vi "Keith 7001 Digital Out Setup.vi"(1 "channel 4 polarity":bool=TRUE, 2 "channel 4 status":bool, 3 "channel 3 polarity":bool=TRUE, 4 "channel 3 status":bool, 5 "channel 2 polarity":bool=TRUE, 6 "channel 2 status":bool, 7 "error in":T1, 8 "channel 1 polarity":bool=TRUE, 9 "channel 1 status":bool, 10 "GPIB address":string="7") -> (0 "error out":T1)   [LabVIEW 2019]
doc: "This VI for the Keithley 7001 Switch System sets the state and polarity (active high/low) of the four digital output ports."
panel:
  # "on\noff"
  # "active high\nactive low"
  # "on\noff"
  # "active high\nactive low"
  # "on\noff"
  # "active high\nactive low"
  # "on\noff"
  # "active high\nactive low"
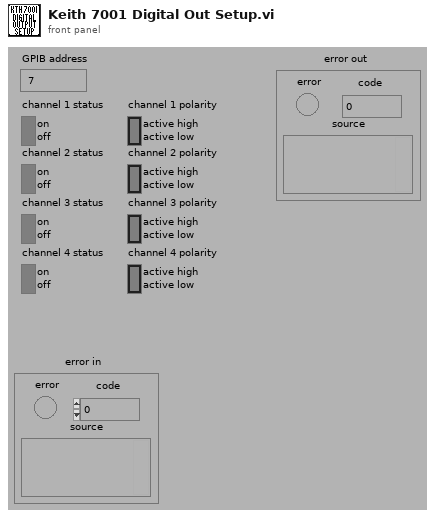
[diagram p1: front panel]
types:
  T1 = cluster{"error":bool, "code":i32, "source":string}
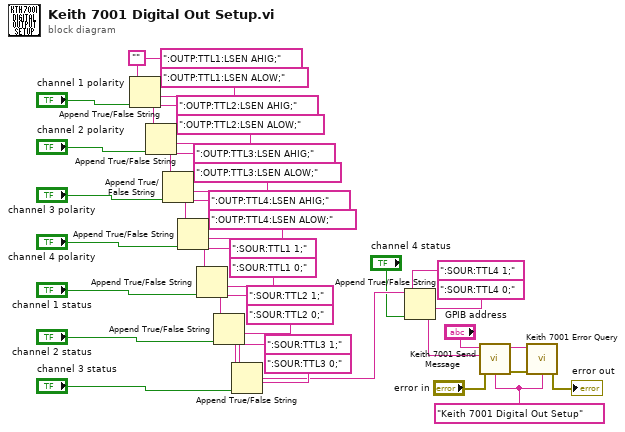
[diagram p0: block diagram]
diagram:
  w2 = "Keith 7001 Digital Out Setup"
  n1 = Append True/False String(1:"channel 1 polarity", 2:":OUTP:TTL1:LSEN ALOW;", 3:":OUTP:TTL1:LSEN AHIG;", 4:"") -> (0:w8:string)
  n2 = Append True/False String(1:"channel 2 polarity", 2:":OUTP:TTL2:LSEN ALOW;", 3:":OUTP:TTL2:LSEN AHIG;", 4:w8) -> (0:w7:string)
  n3 = Append True/False String(1:"channel 3 polarity", 2:":OUTP:TTL3:LSEN ALOW;", 3:":OUTP:TTL3:LSEN AHIG;", 4:w7) -> (0:w6:string)
  n4 = Append True/False String(1:"channel 4 polarity", 2:":OUTP:TTL4:LSEN ALOW;", 3:":OUTP:TTL4:LSEN AHIG;", 4:w6) -> (0:w29:string)
  n5 = Append True/False String(1:"channel 1 status", 2:":SOUR:TTL1 0;", 3:":SOUR:TTL1 1;", 4:w29) -> (0:w27:string)
  n6 = Append True/False String(1:"channel 2 status", 2:":SOUR:TTL2 0;", 3:":SOUR:TTL2 1;", 4:w27) -> (0:w22:string)
  n7 = Append True/False String(1:"channel 3 status", 2:":SOUR:TTL3 0;", 3:":SOUR:TTL3 1;", 4:w22) -> (0:w10:string)
  n8 = Append True/False String(1:"channel 4 status", 2:":SOUR:TTL4 0;", 3:":SOUR:TTL4 1;", 4:w10) -> (0:w19:string)
  n9 = call "Keith 7001 Send Message.vi"("address string"="GPIB address", "write buffer"=w19, "source"=w2, "error in"="error in") -> ("address out"=w4:string, "error out"=w3:T1)  [unwired: 2 in, 2 out]
  n10 = call "Keith 7001 Error Query.vi"("GPIB address"=w4, "error in"=w3, "source"=w2) -> ("error out"=→"error out":T1)  [unwired: 2 out]
